vi "Check-setting-conflicts.vi"(7 "Passed? in":bool=TRUE, 8 "error in":errorcluster, 11 "Data ref. in":refnum<data-value>) -> (0 "error IO":errorcluster, 3 "Data ref.":refnum<data-value>, 5 "Passed?":bool)   [LabVIEW 2013, in "CameraVision.lvlib" / "CV-Main.lvclass"]
doc: "Check for conflicts between the values of different parameters.\nA separate and custom error message is shown for each detected conflict.\n\nThe current checks are:\n- Required values the temperature field calculation.\n- Required values for the temperature value field calculation.\n- Required values for the calculation of the characteristic map.\n- Required values for the calculation of spatial melt pool characteristics."
uses:
  CV-Main.lvclass
  UI/Popup-messages.ctl
  CV-Main.lvclass/CV-Main.ctl
  Read Acquis params.vi
  Read Analysis params.vi
  Read Config params.vi
  Read Correct params.vi
  Read Filter params.vi
  Read Mapping params.vi
  Read Storage params.vi
  Read Temperature params.vi
  Acquisition/CV-Acquisition.lvclass
  Analysis/CV-Analysis.lvclass
  Configuration/CV-Configuration.lvclass
  Correction/CV-Correction.lvclass
  Filter/CV-Filter.lvclass
  Mapping/CV-Mapping.lvclass
  Storage/CV-Storage.lvclass
  Temperature/CV-Temperature.lvclass
  UI/CV-UI.lvclass
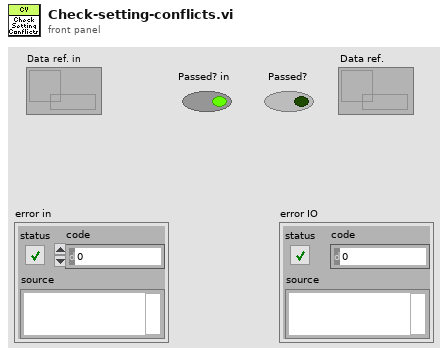
[diagram p1: front panel]
types:
  T1 = typedef "CameraVision.lvlib/CV-UI.lvclass/Popup-messages.ctl" = enum16{"Error-Black image", "Error-Camera config file", "Error-Camera connect", "Error-Grabber init", "Error-Camera setting", "Error-Image offset", "Error-Image import", "Error-Settings file not exist", "Error-Timing source", "Conflict-Filters", "Conflict-Map", "Conflict-Framerate", "Conflict-Charact", "Conflict-Temperature field", "Conflict-Temperature value", "Conflict-Storage-Binary image", "Conflict-Storage-Corrected image", "Conflict-Storage-Map", "Conflict-Storage-Charact", "Conflict-Storage-Temperature field", "Conflict-Storage-Temperature value", "Warning-File exist", "Warning-Parameter reset", "Warning-User cancel", "Info-Images imported"}
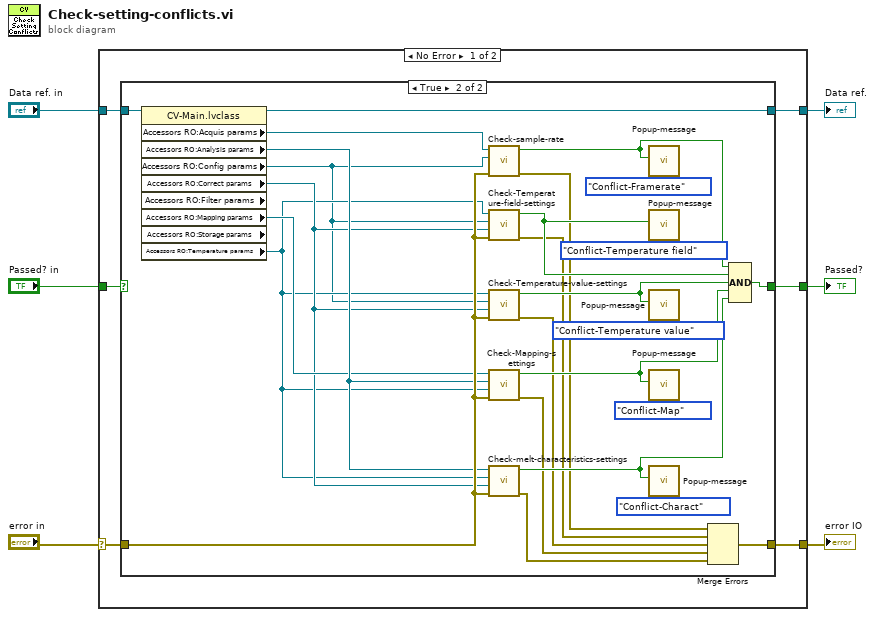
[diagram p0: block diagram]
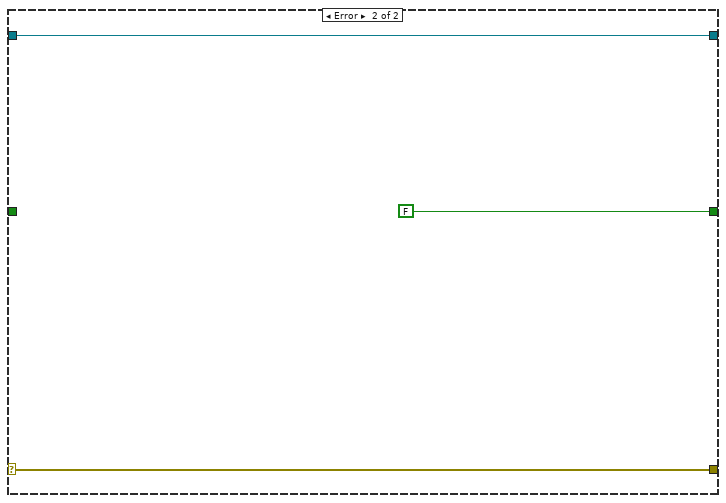
[diagram p3: hidden frame]
diagram:
  n1 = case shown="No Error" "error in" {
    selector: "error in" -> [w10 w43]
    tunnel: [w9 w43] -> w5
    tunnel: [w12 FALSE] -> w6
    tunnel: "Passed? in" -> [w11 _]
    tunnel: "Data ref. in" -> [w8 w42]
    tunnel: [w7 w42] -> w1
    frame No Error {
      n2 = case shown="True" w11 {
        selector: w11 -> [w15 _]
        tunnel: [w15 w41] -> w12
        tunnel: w10 -> [w14 w39]
        tunnel: [w14 w40] -> w9
        tunnel: w8 -> [w13 w38]
        tunnel: [w13 w37] -> w7
        frame False {
        }
        frame True {
          n3 = property class="CV-Main.lvclass" props=["Accessors RO:Acquis params", "Accessors RO:Analysis params", "Accessors RO:Config params", "Accessors RO:Correct params", "Accessors RO:Filter params", "Accessors RO:Mapping params", "Accessors RO:Storage params", "Accessors RO:Temperature params"](reference=w38) -> (reference out=w37:refnum<data-value>, "Accessors RO:Acquis params"=w31:refnum<data-value>, "Accessors RO:Analysis params"=w36:refnum<data-value>, "Accessors RO:Config params"=w32:refnum<data-value>, "Accessors RO:Correct params"=w34:refnum<data-value>, "Accessors RO:Mapping params"=w35:refnum<data-value>, "Accessors RO:Temperature params"=w33:refnum<data-value>)  [unwired: 1 in, 3 out]
          n4 = call "Check-sample-rate.vi"("error in"=w39, "Config. params. ref."=w32, "Acquis. params. ref."=w31) -> ("error IO"=w25:errorcluster, "Passed?"=w26:bool)  [unwired: 7 in]
          n5 = call "Check-Temperature-field-settings.vi"("error in"=w39, "Correct. params. ref."=w34, "Config. params. ref."=w32, "Temp. params. ref."=w33) -> ("error IO"=w24:errorcluster, "Passed?"=w27:bool)  [unwired: 6 in]
          n6 = call "Check-Temperature-value-settings.vi"("error in"=w39, "Correct. params. ref."=w34, "Config. params. ref."=w32, "Temp. params. ref."=w33) -> ("error IO"=w23:errorcluster, "Passed?"=w28:bool)  [unwired: 6 in]
          n7 = call "Check-Mapping-settings.vi"("error in"=w39, "Temp. params. ref."=w33, "Analysis params. ref."=w36, "Mapping params. ref."=w35) -> ("error IO"=w22:errorcluster, "Passed?"=w29:bool)  [unwired: 6 in]
          n8 = call "Check-melt-characteristics-settings.vi"("error in"=w39, "Correct. params. ref."=w34, "Temp. params. ref."=w33, "Analysis params. ref."=w36) -> ("error IO"=w21:errorcluster, "Passed?"=w30:bool)  [unwired: 6 in]
          n9 = call "Popup-message.vi"("Message"=Popup-messages."Conflict-Framerate", "Ignore?"=w26) -> ()  [unwired: 9 in, 1 out]
          n10 = call "Popup-message.vi"("Message"=Popup-messages."Conflict-Temperature field", "Ignore?"=w27) -> ()  [unwired: 9 in, 1 out]
          n11 = call "Popup-message.vi"("Message"=Popup-messages."Conflict-Temperature value", "Ignore?"=w28) -> ()  [unwired: 9 in, 1 out]
          n12 = call "Popup-message.vi"("Message"=Popup-messages."Conflict-Map", "Ignore?"=w29) -> ()  [unwired: 9 in, 1 out]
          n13 = call "Popup-message.vi"("Message"=Popup-messages."Conflict-Charact", "Ignore?"=w30) -> ()  [unwired: 9 in, 1 out]
          n14 = Merge Errors(w25, w24, w23, w22, w21) -> (w40:errorcluster)
          n15 = Compound Arithmetic op=AND(w26, w27, w28, w29, w30) -> (w41:bool)
        }
      }
    }
    frame Error {
    }
  }
  "Passed?" <- w6
  "error IO" <- w5
  "Data ref." <- w1
